vi "Config Notifier Controller.vi"(4 "Paras In 2":variant, 6 "Paras In":variant, 7 "Node Controller Factory In":refnum<class "Node Controller Factory.lvclass">, 8 "error in (no error)":errorcluster, 9 "Notifier Type":refnum<class "Notifier.lvclass">, 10 "Root Actor In":refnum<class "Root Actor.lvclass">, 11 "System Modules Factory in":refnum<class "System Modules Factory.lvclass">) -> (0 "error out":errorcluster, 2 "Root Actor Out":refnum<class "Root Actor.lvclass">, 3 "System Modules Factory out":refnum<class "System Modules Factory.lvclass">, 5 "Node Controller Factory out":refnum<class "Node Controller Factory.lvclass">)   [LabVIEW 2024, in "System Modules Factory.lvclass"]
uses:
  System Modules Factory.lvclass
  Actor/Root Actor/Root Actor.lvclass
  Node Controller Factory/Node Controller Factory.lvclass
  Actor Assistant/Notifier/Notifier.lvclass
  System Modules Factory.lvclass/System Modules Factory.ctl
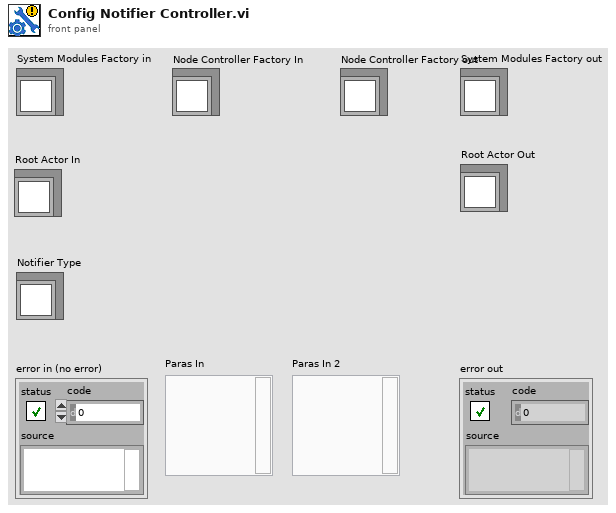
[diagram p1: front panel]
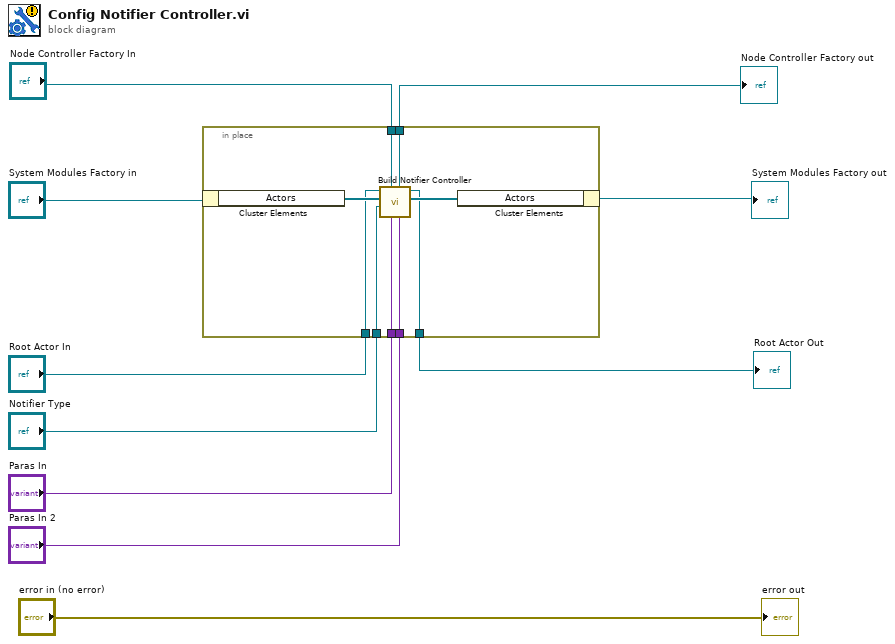
[diagram p0: block diagram]
diagram:
  n1 = in-place {
    in-place-border: "Root Actor In" -> [w17]
    in-place-border: [w16] -> w6
    in-place-border: "Node Controller Factory In" -> [w15]
    in-place-border: [w14] -> w4
    in-place-border: "Paras In" -> [w13]
    in-place-border: "Paras In 2" -> [w12]
    in-place-border: "Notifier Type" -> [w11]
    n2 = in-place-cluster #1("System Modules Factory in") -> ("Actors"=w19:refnum<class "System Actor.lvclass">[])
    n3 = call-dynamic "Build Notifier Controller.vi"("Paras In 2"=w12, "Paras In"=w13, "Node Controller Factory in"=w15, "Notifier Type"=w11, "System Actors In"=w19, "Root Actor In"=w17) -> ("System Actors Out"=w18:refnum<class "System Actor.lvclass">[], "Root Actor Out"=w16:refnum<class "Root Actor.lvclass">, "Node Controller Factory out"=w14:refnum<class "Node Controller Factory.lvclass">)  [unwired: 2 in, 1 out]
    n4 = in-place-cluster #1("Actors"=w18) -> (→"System Modules Factory out":refnum<class "System Modules Factory.lvclass">)
  }
  "Root Actor Out" <- w6
  "Node Controller Factory out" <- w4
  "error out" <- "error in (no error)"
